vi "Destroy User Event - Stop.vi"(8 "error in":errorcluster, 11 "User Events":T1) -> (0 "error out":errorcluster)   [LabVIEW 2019, in "User Events.lvlib"]
doc: "Destroy the user event, even if there is an incoming error."
uses:
  User Events.lvlib
  User Events Typedef.ctl
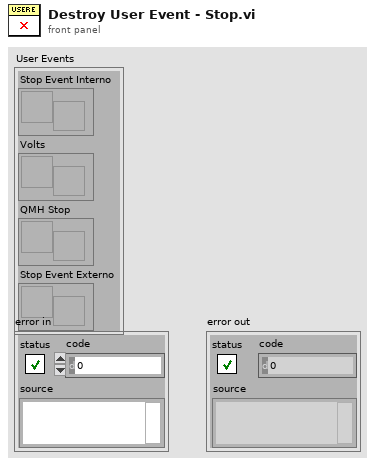
[diagram p1: front panel]
types:
  T1 = typedef "User Events.lvlib/User Events Typedef.ctl" = cluster{"Stop Event Interno":refnum<user-event>, "Volts":refnum<user-event>, "QMH Stop":refnum<user-event>, "Stop Event Externo":refnum<user-event>}
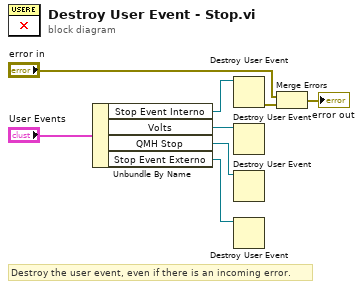
[diagram p0: block diagram]
diagram:
  # "Destroy the user event, even if there is an incoming error."
  n1 = Unbundle By Name("User Events") -> ("Stop Event Interno"=w4:refnum<user-event>, "Volts"=w3:refnum<user-event>, "QMH Stop"=w2:refnum<user-event>, "Stop Event Externo"=w1:refnum<user-event>)
  n2 = Destroy User Event(user event=w4) -> (error out=w8:errorcluster)  [unwired: 1 in]
  n3 = Destroy User Event(user event=w3) -> ()  [unwired: 1 in, 1 out]
  n4 = Destroy User Event(user event=w2) -> ()  [unwired: 1 in, 1 out]
  n5 = Destroy User Event(user event=w1) -> ()  [unwired: 1 in, 1 out]
  n6 = Merge Errors("error in", w8) -> (→"error out":errorcluster)
